vi "SCCSup Help State.vi"(11 "help ref":refnum<vi>) -> (3 "lvdialog path":path)   [LabVIEW 2017]
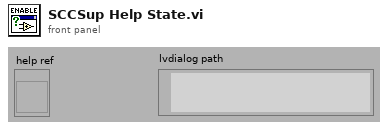
[diagram p1: front panel]
types:
  T1 = enum32{"invalid app kind", "Development System", "Run Time System", "Student Edition", "Embedded LabVIEW", "Evaluation", "Custom"}
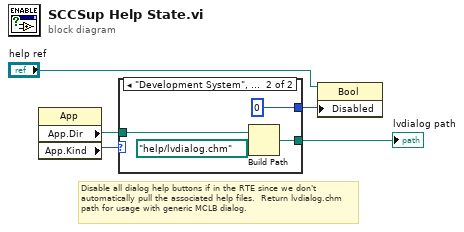
[diagram p0: block diagram]
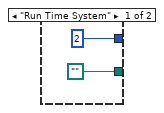
[diagram p2: hidden frame]
diagram:
  # "Disable all dialog help buttons if in the RTE since we don't automatically pull the associated help files.  Return lvdialog.chm path for usage with generic MCLB dialog."
  n1 = property class="App"() -> ("App.Dir"=w4:path, "App.Kind"=w5:T1)  [unwired: 2 in, 2 out]
  n2 = case shown="\"Development System\", Default" w5 {
    tunnel: [u8 2 ("Disabled") u8 0 ("Disabled")] -> w1
    tunnel: w4 -> [_ w9]
    tunnel: [path "" w8] -> w3
    frame "Run Time System" {
    }
    frame "Development System", Default {
      n3 = Build Path(base path=w9, name or relative path=path "help/lvdialog.chm" ("Path to the help file")) -> (appended path=w8:path)
    }
  }
  "lvdialog path" <- w3
  n4 = property class="Bool"(reference="help ref", "Disabled"=w1) -> ()  [unwired: 1 in, 2 out]
